vi "Create Log.vi"(6 "End Cycle?":bool, 7 "Not First Run?":bool, 8 "Error in":errorcluster, 9 "Stop Initiated?":bool, 11 "Log Input Data":T2={"Index Start Time"=timestamp(0 s since 1904-01-01), "Auto Times"={"Index Time"=0, "TF Time"=0, "Insertion Time"=0, "Cutting Time"=0, "PF Time"=0, "Meas. Time"=0, "Reject Time"=0, "P&P Time"=0}, "Tubes Present"=[FALSE, FALSE, FALSE, FALSE], "Reject Pallets"={"Reject 1"=FALSE, "Reject 2"=FALSE, "Reject 3"=FALSE, "Reject 4"=FALSE}, "Measurements"={"1"=0.0, "2"=0.0, "3"=0.0, "4"=0.0}}) -> (2 "Auto Stats":T3)   [LabVIEW 2021]
uses:
  support/Controls/Auto Stats.ctl
  Controls/Auto Times.ctl
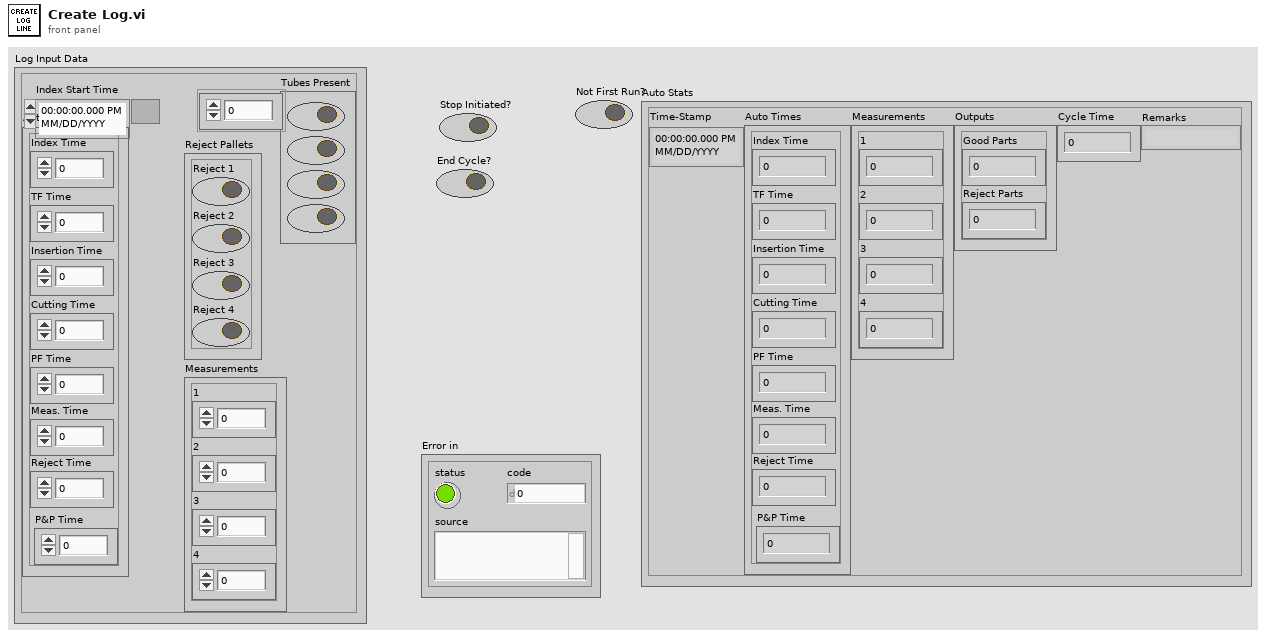
[diagram p1: front panel]
types:
  T1 = typedef "Auto Times.ctl" = cluster{"Index Time":u32, "TF Time":u32, "Insertion Time":u32, "Cutting Time":u32, "PF Time":u32, "Meas. Time":u32, "Reject Time":u32, "P&P Time":u32}
  T2 = cluster{"Index Start Time":timestamp, "Auto Times":T1, "Tubes Present":bool[], "Reject Pallets":cluster{"Reject 1":bool, "Reject 2":bool, "Reject 3":bool, "Reject 4":bool}, "Measurements":cluster{"1":dbl, "2":dbl, "3":dbl, "4":dbl}}
  T3 = typedef "Auto Stats.ctl" = cluster{"Time-Stamp":timestamp, "Auto Times":T1, "Measurements":cluster{"1":dbl, "2":dbl, "3":dbl, "4":dbl}, "Outputs":cluster{"Good Parts":u32, "Reject Parts":u32}, "Cycle Time":dbl, "Remarks":string}
  T4 = cluster{"Reject 1":bool, "Reject 2":bool, "Reject 3":bool, "Reject 4":bool}
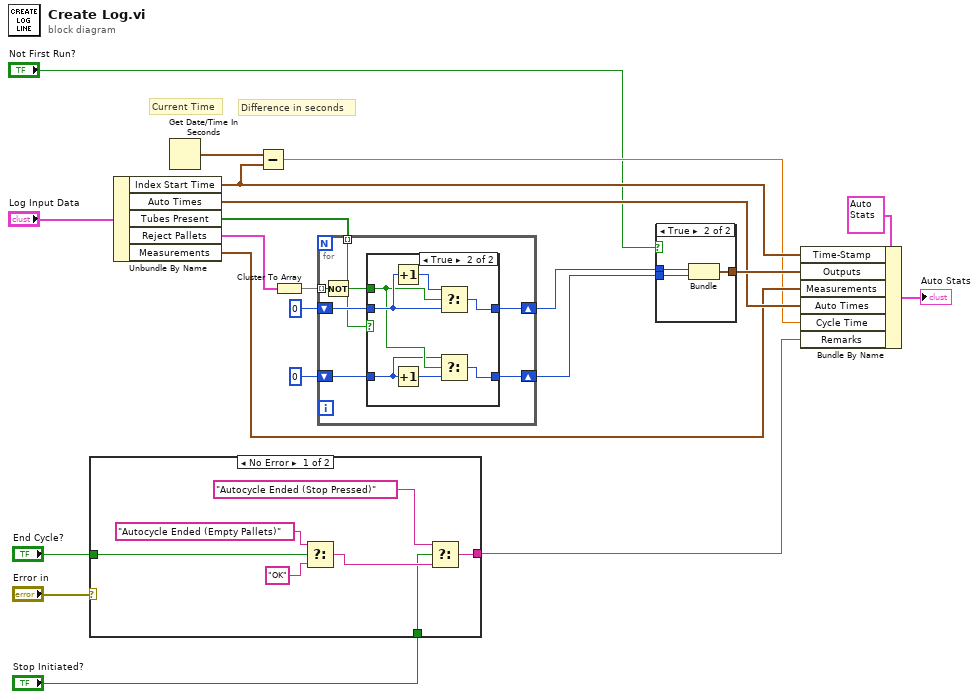
[diagram p0: block diagram]
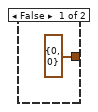
[diagram p2: hidden frame]
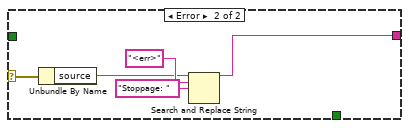
[diagram p3: hidden frame]
diagram:
  # "Difference in seconds"
  # "Current Time"
  n1 = case shown="No Error" "Error in" {
    selector: "Error in" -> [_ w31]
    tunnel: [w24 w30] -> w8
    tunnel: "End Cycle?" -> [w26 _]
    tunnel: "Stop Initiated?" -> [w22 _]
    frame No Error {
      n2 = Select(t="Autocycle Ended (Empty Pallets)" ("result string"), s=w26, f="OK" ("result string")) -> (s? t:f=w25:string)
      n3 = Select(t="Autocycle Ended (Stop Pressed)" ("result string"), s=w22, f=w25) -> (s? t:f=w24:string)
    }
    frame Error {
      n4 = Unbundle By Name(w31) -> ("source"=w32:string)
      n5 = Search and Replace String(input string=w32, search string="<err>", replace string="Stoppage: " ("replace string (\"\")")) -> (result string=w30:string)  [unwired: 5 in, 3 out]
    }
  }
  n6 = Unbundle By Name("Log Input Data") -> ("Index Start Time"=w14:timestamp, "Auto Times"=w13:T1, "Tubes Present"=w2:bool[], "Reject Pallets"=w12:T4, "Measurements"=w11:cluster{"1":dbl, "2":dbl, "3":dbl, "4":dbl})
  n7 = Get Date/Time In Seconds() -> (seconds since 1Jan1904=w16:timestamp)
  n8 = Subtract(x=w16, y=w14) -> (x-y=w10:dbl)
  n9 = Cluster To Array(cluster=w12) -> (array=w21:bool[])
  n10 = for {
    tunnel: w21 -> [w37] mode=indexing
    shift-right: [w40] -> w4
    shift-left: u32 0 -> [w39]
    shift-right: [w38] -> w3
    shift-left: u32 0 -> [w36]
    tunnel: w2 -> [w35] mode=indexing
    n11 = Not(x=w37) -> (.not. x?=w34:bool)
    n12 = case shown="True" w35 {
      tunnel: [w42 w49] -> w40
      tunnel: w39 -> [w42 w48]
      tunnel: [w41 w45] -> w38
      tunnel: w34 -> [_ w44]
      tunnel: w36 -> [w41 w43]
      frame False {
      }
      frame True {
        n13 = Increment(x=w48) -> (x+1=w47:u32)
        n14 = Increment(x=w43) -> (x+1=w46:u32)
        n15 = Select(t=w47, s=w44, f=w48) -> (s? t:f=w49:u32)
        n16 = Select(t=w43, s=w44, f=w46) -> (s? t:f=w45:u32)
      }
    }
  }
  n17 = case shown="True" "Not First Run?" {
    tunnel: [cluster{u32, u32} {0, 0} w53] -> w18
    tunnel: w4 -> [_ w52]
    tunnel: w3 -> [_ w51]
    frame False {
    }
    frame True {
      n18 = Bundle(w52, w51) -> (w53:cluster{u32, u32})  [unwired: 1 in]
    }
  }
  n19 = Bundle By Name(cluster=T3 {"Time-Stamp"=timestamp(0 s since 1904-01-01), "Auto Times"={"Index Time"=0, "TF Time"=0, "Insertion Time"=0, "Cutting Time"=0, "PF Time"=0, "Meas. Time"=0, "Reject Time"=0, "P&P Time"=0}, "Measurements"={"1"=0.0, "2"=0.0, "3"=0.0, "4"=0.0}, "Outputs"={"Good Parts"=0, "Reject Parts"=0}, "Cycle Time"=0.0, "Remarks"=""} ("Auto Stats"), "Time-Stamp"=w14, "Outputs"=w18, "Measurements"=w11, "Auto Times"=w13, "Cycle Time"=w10, "Remarks"=w8) -> (→"Auto Stats":T3)
